vi "stop sign queue.vi"(7 "Action":T1=enum."Enqueue", 8 "error in (no error)":errorcluster, 9 "stop in":bool=TRUE, 10 "time out":i32=100) -> (0 "error out":errorcluster, 1 "stop out":bool, 2 "Empty?":bool, 3 "timed out?":bool)   [LabVIEW 2018]
uses:
  SerialSectOCT_1217/SerialSectOCT/Software/General/Controls/Queue Manager Actions.ctl
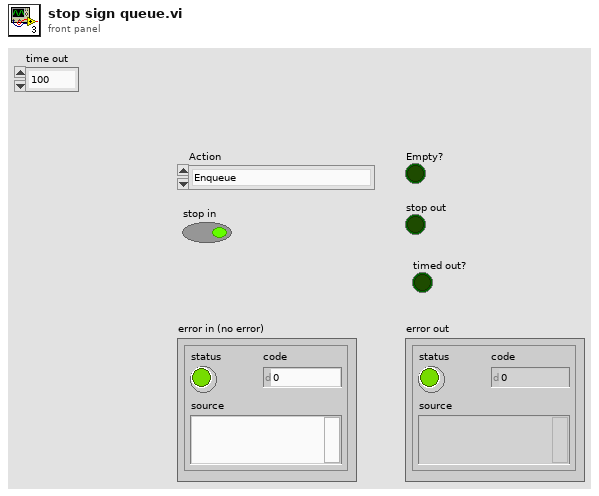
[diagram p1: front panel]
types:
  T1 = typedef "Queue Manager Actions.ctl" = enum16{"Init", "Enqueue", "Enqueue All", "Preview Queue", "Dequeue", "Get Status", "Flush Queue", "Flush All Queues", "Release All Queues", "Release Queue", "Enqueue at Opposite End"}
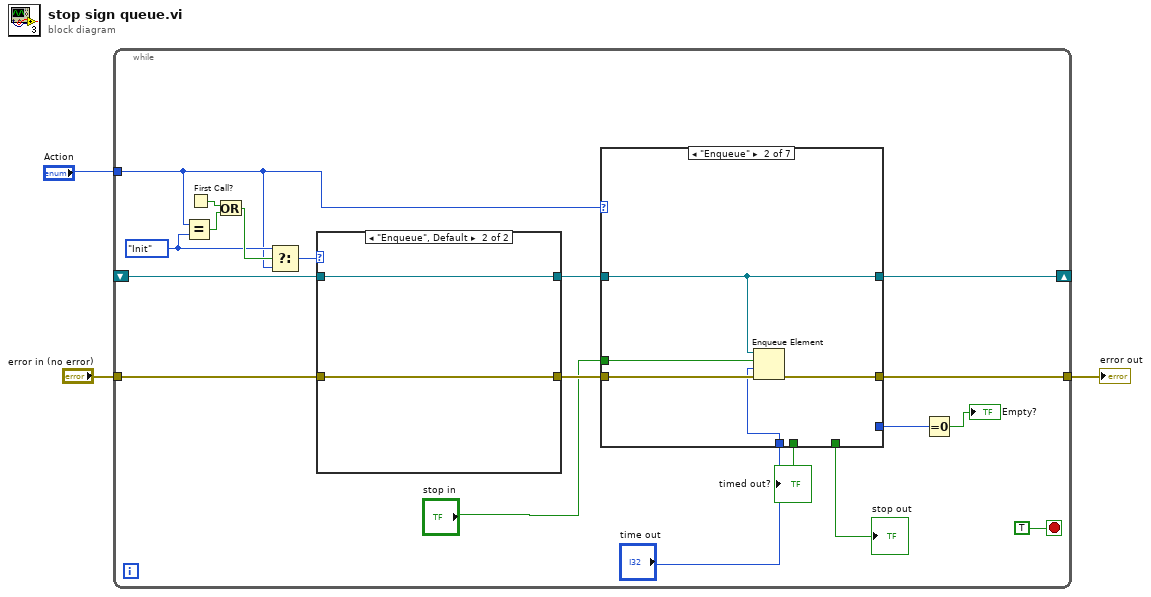
[diagram p0: block diagram]
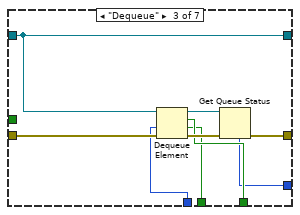
[diagram p3: hidden frame]
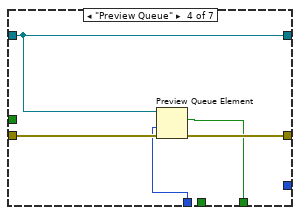
[diagram p4: hidden frame]
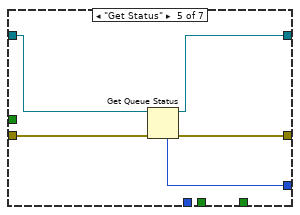
[diagram p5: hidden frame]
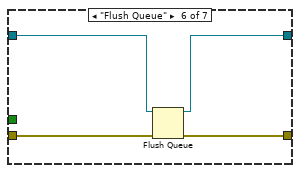
[diagram p6: hidden frame]
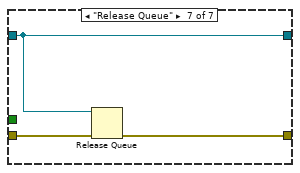
[diagram p7: hidden frame]
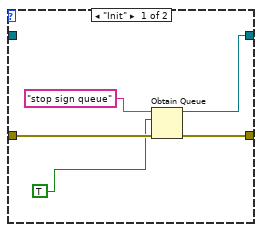
[diagram p8: hidden frame]
diagram:
  n1 = while {
    tunnel: "Action" -> [w10]
    tunnel: "error in (no error)" -> [w17]
    tunnel: [w16] -> w1
    shift-right: [w12] -> _
    shift-left: _ -> [w11]
    stop <- TRUE stop-if-true
    w19 = Queue_Manager_Actions."Init"
    n2 = Equal?(x=w10, y=w19) -> (x = y?=w21:bool)
    n3 = First Call?() -> (First Call?: T/F=w22:bool)
    n4 = Or(x=w22, y=w21) -> (x .or. y?=w20:bool)
    n5 = Select(t=w19, s=w20, f=w10) -> (s? t:f=w18:T1)
    n6 = case shown="\"Enqueue\", Default" w18 {
      tunnel: [w60 w61] -> w14
      tunnel: w17 -> [w59 w62]
      tunnel: [w58 w62] -> w15
      tunnel: w11 -> [_ w61]
      frame "Init" {
        n7 = Obtain Queue(name (unnamed)="stop sign queue" ("queue name"), element data type=TRUE, error in (no error)=w59) -> (queue out=w60:refnum<queue>, error out=w58:errorcluster)  [unwired: 2 in, 1 out]
      }
      frame "Enqueue", Default {
      }
    }
    n8 = case shown="\"Enqueue\"" w10 {
      tunnel: w14 -> [w23 w25 w33 w40 w46 w50 w53]
      tunnel: [w24 w28 w35 w42 w47 w51 w54] -> w16
      tunnel: w15 -> [w24 w29 w38 w43 w48 w52 w55]
      tunnel: [w23 w25 w33 w40 w45 w49 w53] -> w12
      tunnel: "time out" -> [_ w27 w36 w41 _ _ _]
      tunnel: "stop in" -> [_ w26 _ _ _ _ _]
      tunnel: [_ _ w31 _ w44 _ _] -> w7
      tunnel: [_ _ w32 w39 _ _ _] -> w6
      tunnel: [_ _ w30 _ _ _ _] -> w5
      frame "Init", Default {
      }
      frame "Enqueue" {
        n9 = Enqueue Element(queue=w25, element=w26, timeout in ms (-1)=w27, error in (no error)=w29) -> (error out=w28:errorcluster)  [unwired: 2 out]
      }
      frame "Dequeue" {
        n10 = Dequeue Element(queue=w33, timeout in ms (-1)=w36, error in (no error)=w38) -> (queue out=w34:refnum<queue>, element=w32:bool, timed out?=w30:bool, error out=w37:errorcluster)
        n11 = Get Queue Status(queue=w34, error in (no error)=w37) -> (error out=w35:errorcluster, # elements in queue=w31:i32)  [unwired: 1 in, 6 out]
      }
      frame "Preview Queue" {
        n12 = Preview Queue Element(queue=w40, timeout in ms (-1)=w41, error in (no error)=w43) -> (element=w39:bool, error out=w42:errorcluster)  [unwired: 2 out]
      }
      frame "Get Status" {
        n13 = Get Queue Status(queue=w46, error in (no error)=w48) -> (queue out=w45:refnum<queue>, error out=w47:errorcluster, # elements in queue=w44:i32)  [unwired: 1 in, 5 out]
      }
      frame "Flush Queue" {
        n14 = Flush Queue(queue=w50, error in (no error)=w52) -> (queue out=w49:refnum<queue>, error out=w51:errorcluster)  [unwired: 1 out]
      }
      frame "Release Queue" {
        n15 = Release Queue(queue=w53, error in (no error)=w55) -> (error out=w54:errorcluster)  [unwired: 1 in, 2 out]
      }
    }
    "stop out" <- w6
    "timed out?" <- w5
    n16 = Equal To 0?(x=w7) -> (x = 0?=→"Empty?":bool)
  }
  "error out" <- w1
